vi "Comm String Wait For ACK.vi"(0 "niDTS Comm Telnet in":refnum<class "niDTS Comm Telnet.lvclass">, 5 "ACK":string, 7 "Timeout (ms)":i32, 11 "error in (no error)":errorcluster) -> (4 "niDTS Comm Telnet out":refnum<class "niDTS Comm Telnet.lvclass">, 6 "Response":string, 8 "Sucess":bool, 15 "error out":errorcluster)   [LabVIEW 2015, in "niDTS CommLib.lvlib" / "niDTS Comm Telnet.lvclass"]
doc: "Last Read is populated internally.\n\nLogging must be done by the calling VI."
uses:
  niDTS Comm Telnet.lvclass
  Utility/telnet/NI_InternetTK_Core_VIs.lvlib
  String_class/niDTS Comm String.lvclass
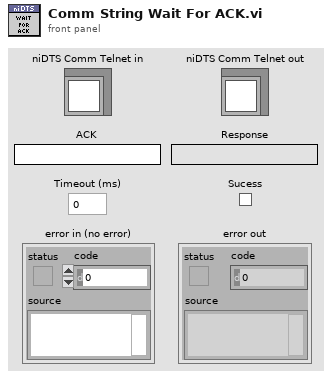
[diagram p1: front panel]
types:
  T1 = typedef "Telnet Session.ctl" = refnum<k1>
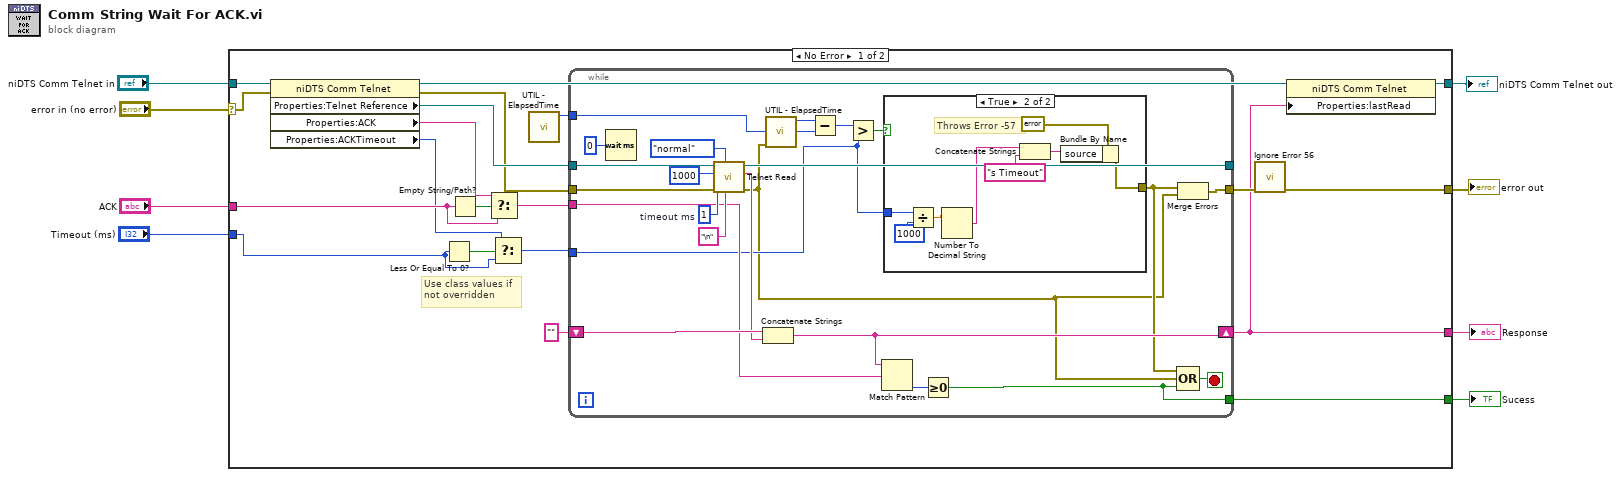
[diagram p0: block diagram]
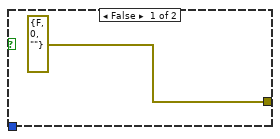
[diagram p2: hidden frame]
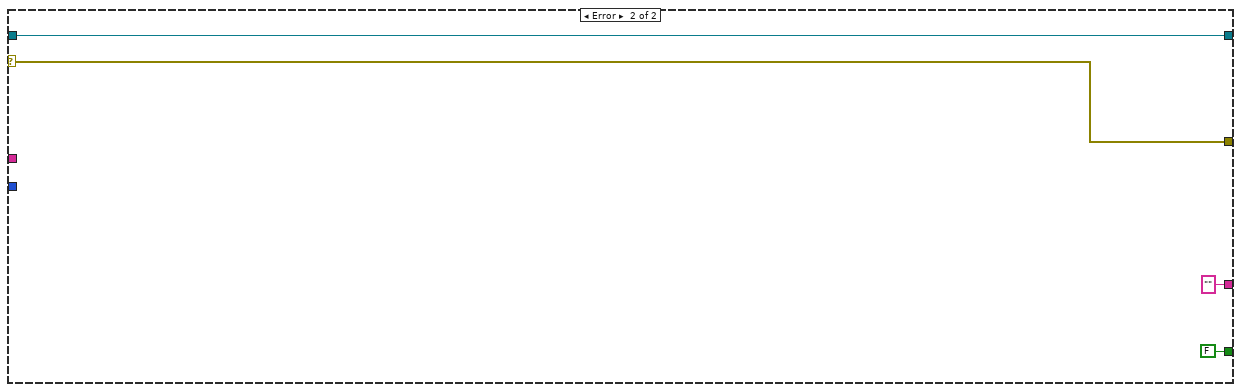
[diagram p3: hidden frame]
diagram:
  n1 = case shown="No Error" "error in (no error)" {
    selector: "error in (no error)" -> [w27 w63]
    tunnel: "niDTS Comm Telnet in" -> [w28 w64]
    tunnel: "ACK" -> [w25 _]
    tunnel: "Timeout (ms)" -> [w22 _]
    tunnel: [w10 "" ("String in")] -> w4
    tunnel: [w14 w63] -> w3
    tunnel: [w11 w64] -> w2
    tunnel: [w13 FALSE] -> w1
    frame No Error {
      # "Use class values if \nnot overridden"
      n2 = property class="niDTS Comm Telnet"(reference=w28, error in=w27) -> (reference out=w12:refnum<class "niDTS Comm Telnet.lvclass">, error out=w19:errorcluster, "Properties:Telnet Reference"=w20:T1, "Properties:ACK"=w24:string, "Properties:ACKTimeout"=w21:i32)
      n3 = Less Or Equal To 0?(x=w22) -> (x <= 0?=w23:bool)
      n4 = Empty String/Path?(string/path=w25) -> (empty?=w26:bool)
      n5 = Select(t=w24, s=w26, f=w25) -> (s? t:f=w17:string)
      n6 = Select(t=w21, s=w23, f=w22) -> (s? t:f=w18:i32)
      n7 = call "UTIL - ElapsedTime.vi"() -> ("ms value"=w9:u32)  [unwired: 9 in, 2 out]
      n8 = while {
        tunnel: [w35] -> w15
        tunnel: [w41] -> _
        shift-right: [w44] -> w10
        shift-left: "" ("String in") -> [w48]
        tunnel: w20 -> [w47]
        tunnel: w19 -> [w46]
        tunnel: w17 -> [w43]
        tunnel: w9 -> [w38]
        tunnel: w18 -> [w32]
        tunnel: [w29] -> w13
        stop <- w42 stop-if-true
        w50 = 1  # timeout ms
        n9 = Wait (ms)(milliseconds to wait=u32 0) -> ()  [unwired: 1 out]
        n10 = call "Telnet Read.vi"("line separator"="\n", "read mode (normal)"=enum16{"normal", "line", "buffered"}."normal", "error in (no error)"=w46, "timeout ms (25000)"=w50, "bytes to read"=1000, "telnet connection"=w47) -> ("error out"=w30:errorcluster, "data out"=w33:string, "telnet connection out"=w41:T1)  [unwired: 1 in]
        n11 = Concatenate Strings(w48, w33) -> (w44:string)
        n12 = call "UTIL - ElapsedTime.vi"("error in"=w30) -> ("ms value"=w39:u32)  [unwired: 8 in, 2 out]
        n13 = Subtract(x=w39, y=w38) -> (x-y=w37:u32)
        n14 = Greater?(x=w37, y=w32) -> (0:w36:bool)
        n15 = Match Pattern(string=w44, regular expression=w43) -> (offset past match=w45:i32)  [unwired: 1 in, 3 out]
        n16 = case shown="True" w36 {
          tunnel: [errorcluster {"status"=FALSE, "code"=0, "source"=""} ("error constant") w54] -> w34
          tunnel: w32 -> [_ w60]
          frame False {
          }
          frame True {
            # "Throws Error -57"
            n17 = Divide(x=w60, y=1000) -> (x/y=w58:dbl)
            n18 = Number To Decimal String(number=w58) -> (decimal integer string=w53:string)  [unwired: 1 in]
            n19 = Concatenate Strings(w53, "s Timeout") -> (w55:string)
            n20 = Bundle By Name(cluster=errorcluster {"status"=TRUE, "code"=-57, "source"="40 s Timeout"} ("error constant"), "source"=w55) -> (w54:errorcluster)
          }
        }
        n21 = Greater Or Equal To 0?(x=w45) -> (x >= 0?=w29:bool)
        n22 = Compound Arithmetic op=OR(w34, w30, w29) -> (w42:bool)
        n23 = Merge Errors(w34, w30) -> (w35:errorcluster)
      }
      n24 = call "Ignore Error 56.vi"("error in (no error)"=w15) -> ("error out"=w14:errorcluster)  [unwired: 10 in]
      n25 = property class="niDTS Comm Telnet"(reference=w12, "Properties:lastRead"=w10) -> (reference out=w11:refnum<class "niDTS Comm Telnet.lvclass">)  [unwired: 1 in, 1 out]
    }
    frame Error {
    }
  }
  "error out" <- w3
  "niDTS Comm Telnet out" <- w2
  "Response" <- w4
  "Sucess" <- w1
